vi "test BroadcastRegistry2.vi"() -> ()   [LabVIEW 2017]
uses:
  user.lib/_NEVSTOP/Communicable State Machine(CSM)/_Support/FGV-BroadcastRegistry/Operation-BroadcastRegistry.ctl
  user.lib/_NEVSTOP/Communicable State Machine(CSM)/Communicable State Machine.lvlib
panel:
  out "response message":string[](array[string])
  out "response message":string[](array[string])
  out "response message":string[](array[string])
  out "response message":string[](array[string])
  out "response message":string[](array[string])
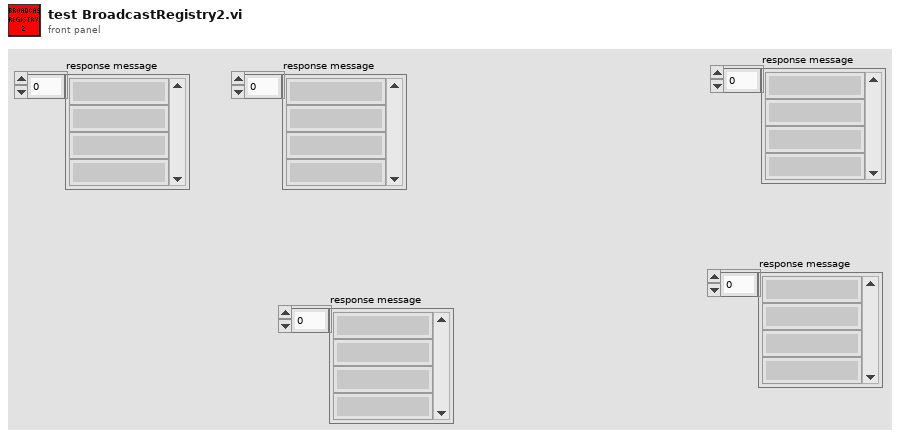
[diagram p1: front panel]
types:
  T1 = typedef "Communicable State Machine.lvlib/Operation-BroadcastRegistry.ctl" = enum16{"Delete Source Module", "Delete Target Module", "Remove Module", "Register", "Unregister", "Check"}
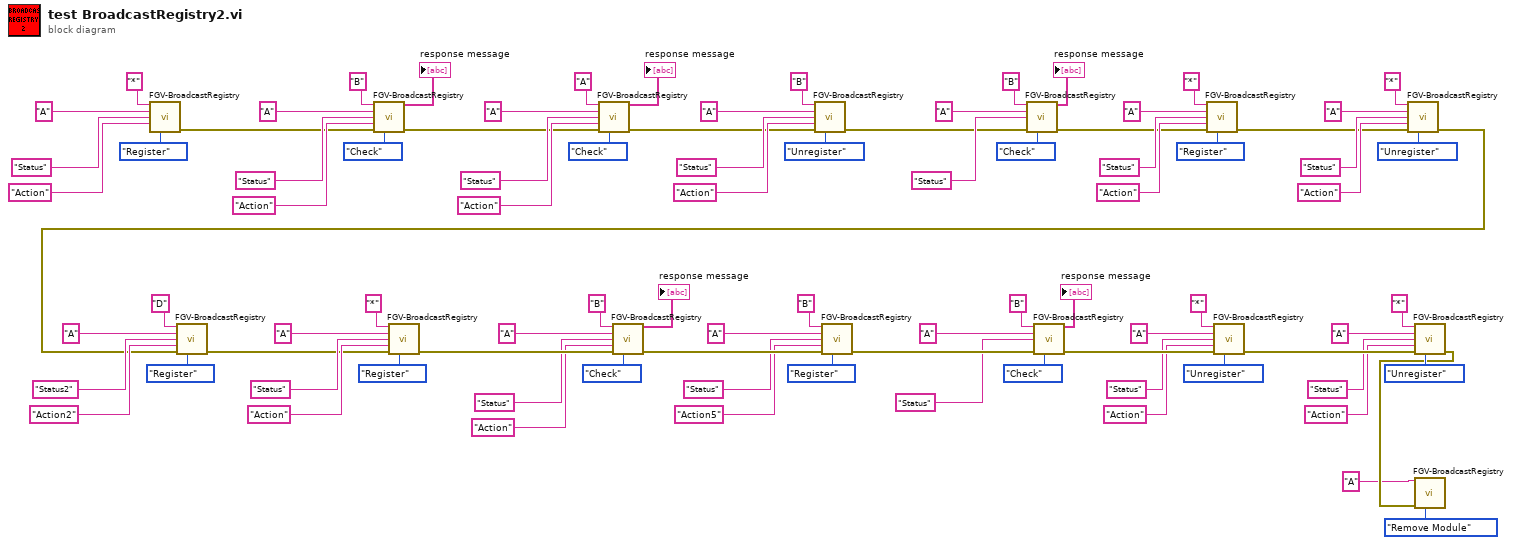
[diagram p0: block diagram]
diagram:
  n1 = call "FGV-BroadcastRegistry.vi"("Source"="*", "Target"="A" ("Dest"), "Status"="Status" ("Message"), "API"="Action" ("Response Message In"), "Operation"=Operation-BroadcastRegistry."Register") -> ("Error out"=w79:errorcluster)  [unwired: 9 in, 1 out]
  n2 = call "FGV-BroadcastRegistry.vi"("Source"="B", "Target"="A" ("Dest"), "Status"="Status" ("Message"), "API"="Action" ("Response Message In"), "Error in"=w79, "Operation"=Operation-BroadcastRegistry."Check") -> ("response message"=→"response message":string[], "Error out"=w2:errorcluster)  [unwired: 8 in]
  n3 = call "FGV-BroadcastRegistry.vi"("Source"="A", "Target"="A" ("Dest"), "Status"="Status" ("Message"), "API"="Action" ("Response Message In"), "Error in"=w2, "Operation"=Operation-BroadcastRegistry."Check") -> ("response message"=→"response message":string[], "Error out"=w1:errorcluster)  [unwired: 8 in]
  n4 = call "FGV-BroadcastRegistry.vi"("Source"="B", "Target"="A" ("Dest"), "Status"="Status" ("Message"), "API"="Action" ("Response Message In"), "Error in"=w1, "Operation"=Operation-BroadcastRegistry."Unregister") -> ("Error out"=w67:errorcluster)  [unwired: 8 in, 1 out]
  n5 = call "FGV-BroadcastRegistry.vi"("Source"="B", "Target"="A" ("Dest"), "Status"="Status" ("Message"), "Error in"=w67, "Operation"=Operation-BroadcastRegistry."Check") -> ("response message"=→"response message":string[], "Error out"=w61:errorcluster)  [unwired: 9 in]
  n6 = call "FGV-BroadcastRegistry.vi"("Source"="*", "Target"="A" ("Dest"), "Status"="Status" ("Message"), "API"="Action" ("Response Message In"), "Error in"=w61, "Operation"=Operation-BroadcastRegistry."Register") -> ("Error out"=w55:errorcluster)  [unwired: 8 in, 1 out]
  n7 = call "FGV-BroadcastRegistry.vi"("Source"="*", "Target"="A" ("Dest"), "Status"="Status" ("Message"), "API"="Action" ("Response Message In"), "Error in"=w55, "Operation"=Operation-BroadcastRegistry."Unregister") -> ("Error out"=w13:errorcluster)  [unwired: 8 in, 1 out]
  n8 = call "FGV-BroadcastRegistry.vi"("Source"="D", "Target"="A" ("Dest"), "Status"="Status2" ("Message"), "API"="Action2" ("Response Message In"), "Error in"=w13, "Operation"=Operation-BroadcastRegistry."Register") -> ("Error out"=w12:errorcluster)  [unwired: 8 in, 1 out]
  n9 = call "FGV-BroadcastRegistry.vi"("Source"="*", "Target"="A" ("Dest"), "Status"="Status" ("Message"), "API"="Action" ("Response Message In"), "Error in"=w12, "Operation"=Operation-BroadcastRegistry."Register") -> ("Error out"=w29:errorcluster)  [unwired: 8 in, 1 out]
  n10 = call "FGV-BroadcastRegistry.vi"("Source"="B", "Target"="A" ("Dest"), "Status"="Status" ("Message"), "API"="Action" ("Response Message In"), "Error in"=w29, "Operation"=Operation-BroadcastRegistry."Check") -> ("response message"=→"response message":string[], "Error out"=w36:errorcluster)  [unwired: 8 in]
  n11 = call "FGV-BroadcastRegistry.vi"("Source"="B", "Target"="A" ("Dest"), "Status"="Status" ("Message"), "API"="Action5" ("Response Message In"), "Error in"=w36, "Operation"=Operation-BroadcastRegistry."Register") -> ("Error out"=w42:errorcluster)  [unwired: 8 in, 1 out]
  n12 = call "FGV-BroadcastRegistry.vi"("Source"="B", "Target"="A" ("Dest"), "Status"="Status" ("Message"), "Error in"=w42, "Operation"=Operation-BroadcastRegistry."Check") -> ("response message"=→"response message":string[], "Error out"=w48:errorcluster)  [unwired: 9 in]
  n13 = call "FGV-BroadcastRegistry.vi"("Source"="*", "Target"="A" ("Dest"), "Status"="Status" ("Message"), "API"="Action" ("Response Message In"), "Error in"=w48, "Operation"=Operation-BroadcastRegistry."Unregister") -> ("Error out"=w54:errorcluster)  [unwired: 8 in, 1 out]
  n14 = call "FGV-BroadcastRegistry.vi"("Source"="*", "Target"="A" ("Dest"), "Status"="Status" ("Message"), "API"="Action" ("Response Message In"), "Error in"=w54, "Operation"=Operation-BroadcastRegistry."Unregister") -> ("Error out"=w10:errorcluster)  [unwired: 8 in, 1 out]
  n15 = call "FGV-BroadcastRegistry.vi"("Source"="A" ("Dest"), "Error in"=w10, "Operation"=Operation-BroadcastRegistry."Remove Module") -> ()  [unwired: 11 in, 2 out]
